vi "Cache.Result.Write.vi"(6 "Time (now)":timestamp, 7 "Idx":i32, 8 "error in (no error)":errorcluster, 9 "ProdComp":T1, 10 "Result in":T2) -> (0 "error out":errorcluster, 3 "File":string)   [LabVIEW 2016]
uses:
  Cache.TestSteps.Fglb.ResultData.ctl
  Database/ProdaNG/Controls/ProdaNG.ProcessResult.ctl
  Database/ProdaNG/Controls/ProdaNG.ProcessStepResult.ctl
  Database/ProdaNG/Controls/ProdaNG.TestStepResult.ctl
  Database/ProdaNG/Controls/ProdaNG.TestValueResult.ctl
  Cache.ProductComponent.Data.ctl
  Global/ApplicationGlobal.vi
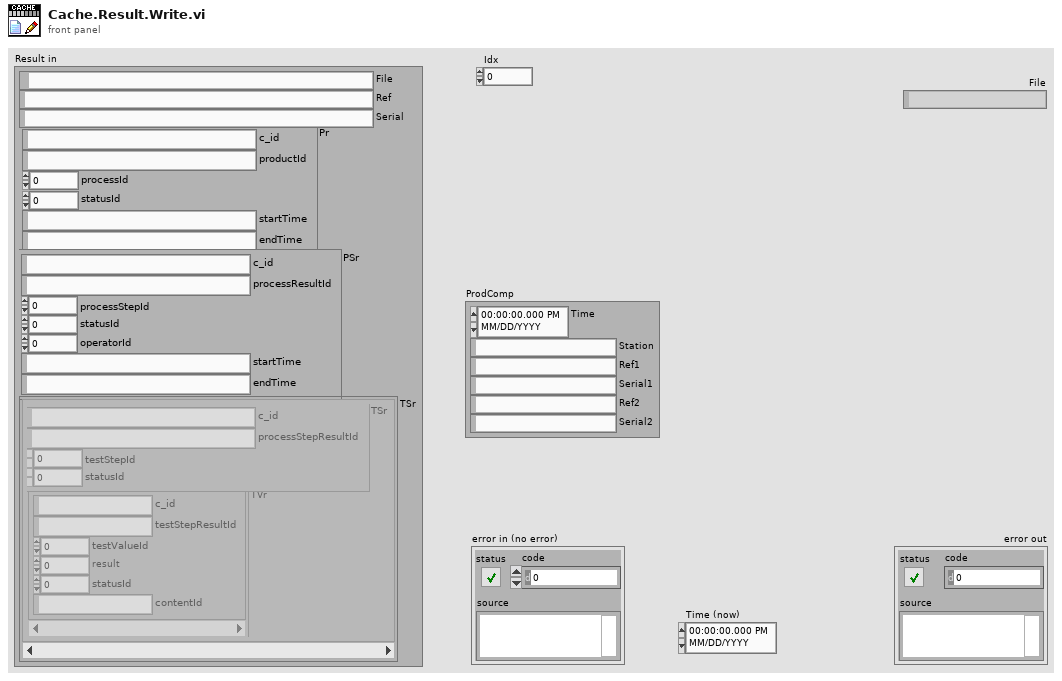
[diagram p1: front panel]
types:
  T1 = typedef "Cache.ProductComponent.Data.ctl" = cluster{"Time":timestamp, "Station":string, "Ref1":string, "Serial1":string, "Ref2":string, "Serial2":string}
  T2 = typedef "Cache.TestSteps.Fglb.ResultData.ctl" = cluster{"File":path, "Ref":string, "Serial":string, "Pr":T3, "PSr":T4, "TSr":cluster{"TSr":T5, "TVr":T6[]}[]}
  T3 = typedef "ProdaNG.ProcessResult.ctl" = cluster{"c_id":string, "productId":string, "processId":i32, "statusId":i32, "startTime":string, "endTime":string}
  T4 = typedef "ProdaNG.ProcessStepResult.ctl" = cluster{"c_id":string, "processResultId":string, "processStepId":i32, "statusId":i32, "operatorId":i32, "startTime":string, "endTime":string}
  T5 = typedef "ProdaNG.TestStepResult.ctl" = cluster{"c_id":string, "processStepResultId":string, "testStepId":i32, "statusId":i32}
  T6 = typedef "ProdaNG.TestValueResult.ctl" = cluster{"c_id":string, "testStepResultId":string, "testValueId":i32, "result":dbl, "statusId":i32, "contentId":string}
  T7 = enum16{"open", "open or create", "create or replace", "create", "open (read-only)"}
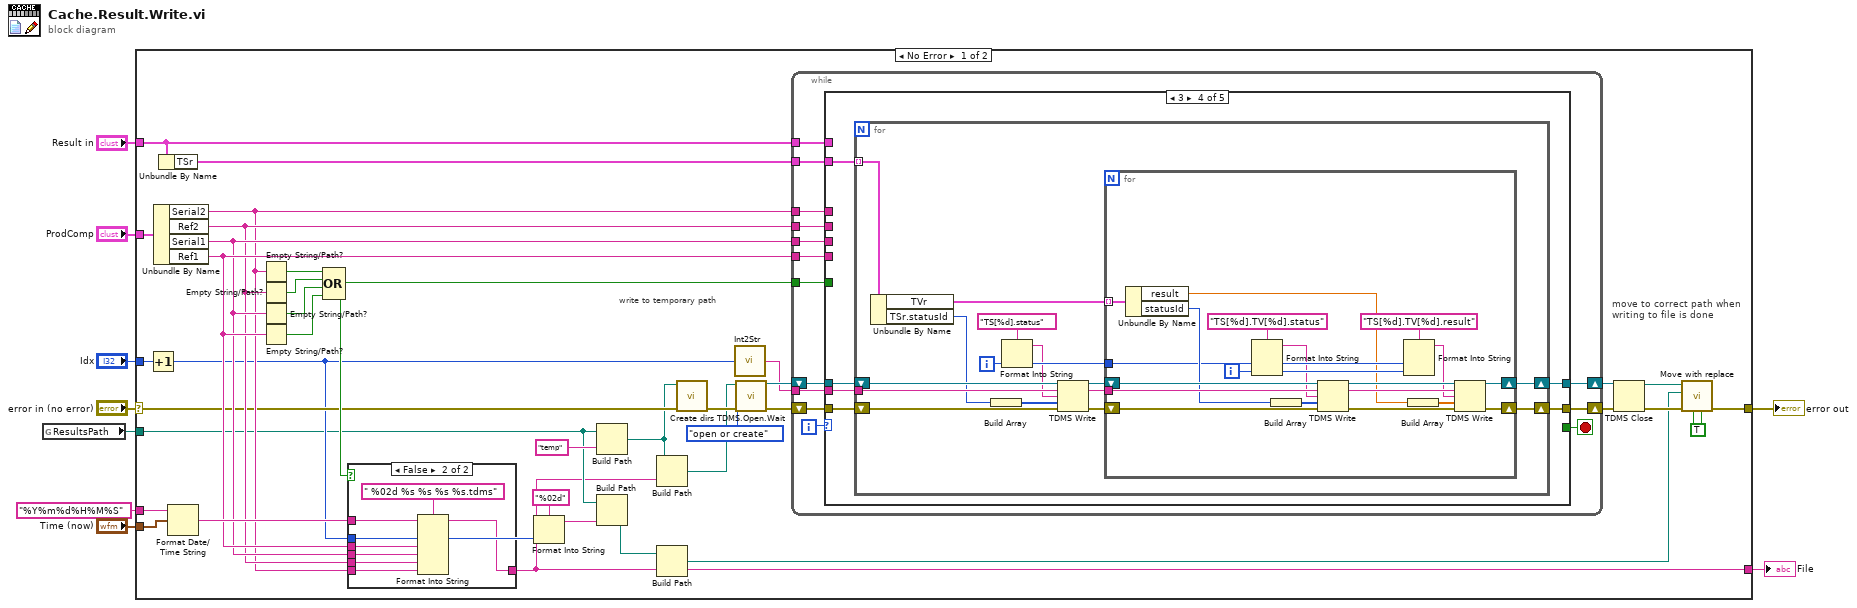
[diagram p0: block diagram]
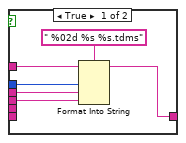
[diagram p2: hidden frame]
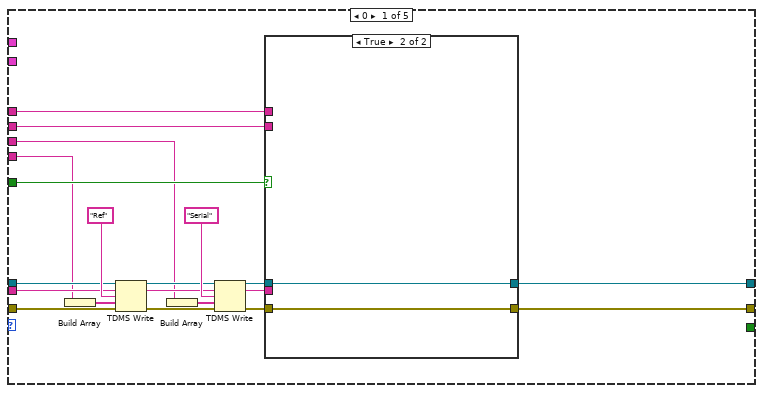
[diagram p3: hidden frame]
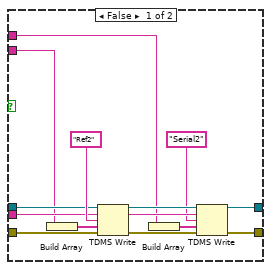
[diagram p4: hidden frame]
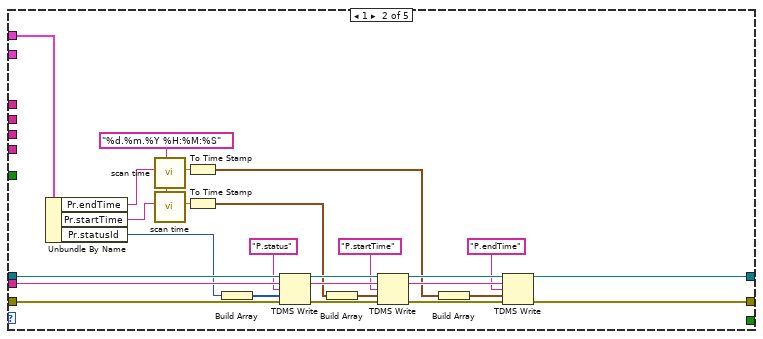
[diagram p5: hidden frame]
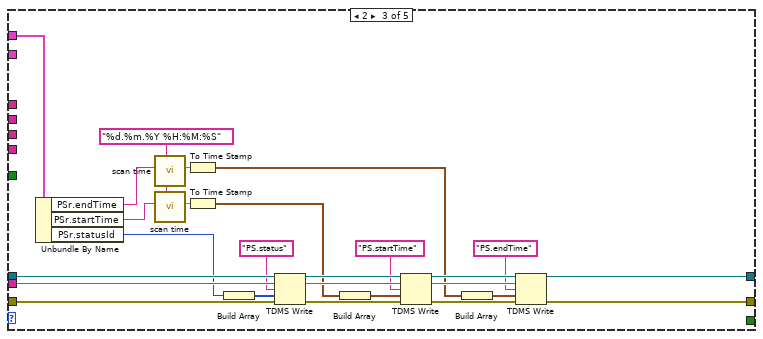
[diagram p6: hidden frame]
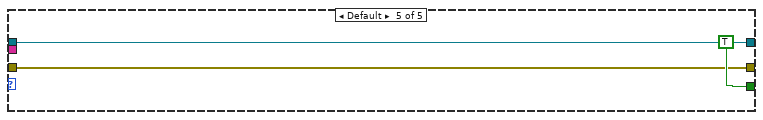
[diagram p7: hidden frame]
diagram:
  n1 = global read "ApplicationGlobal.vi" "ResultsPath"() -> (w4:path)
  n2 = case shown="No Error" "error in (no error)" {
    selector: "error in (no error)" -> [w25 w207]
    tunnel: "Result in" -> [w47 _]
    tunnel: [w20 w207] -> w9
    tunnel: "Idx" -> [w40 _]
    tunnel: "ProdComp" -> [w34 _]
    tunnel: w4 -> [w15 _]
    tunnel: "Time (now)" -> [w32 _]
    tunnel: "%Y%m%d%H%M%S" ("time format string (%c)") -> [w33 _]
    tunnel: [w12 _] -> w1
    frame No Error {
      w11 = TRUE ("create parent dirs (F)")
      # "move to correct path when \nwriting to file is done"
      # "write to temporary path"
      n3 = Increment(x=w40) -> (x+1=w23:i32)
      n4 = Unbundle By Name(w34) -> ("Serial2"=w26:string, "Ref2"=w27:string, "Serial1"=w28:string, "Ref1"=w29:string)
      n5 = Unbundle By Name(w47) -> ("TSr"=w43:cluster{"TSr":T5, "TVr":T6[]}[])
      n6 = Format Date/Time String(time format string (%c)=w33, seconds (now)=w32) -> (date/time string=w31:string)  [unwired: 1 in]
      n7 = Empty String/Path?(string/path=w26) -> (empty?=w38:bool)
      n8 = Empty String/Path?(string/path=w27) -> (empty?=w37:bool)
      n9 = Empty String/Path?(string/path=w28) -> (empty?=w36:bool)
      n10 = Empty String/Path?(string/path=w29) -> (empty?=w35:bool)
      n11 = Compound Arithmetic op=OR(w38, w37, w36, w35) -> (w30:bool)
      n12 = case shown="False" w30 {
        tunnel: [w48 w57] -> w12
        tunnel: w23 -> [w52 w54]
        tunnel: w31 -> [w49 w58]
        tunnel: w29 -> [w51 w60]
        tunnel: w28 -> [w50 w59]
        tunnel: w27 -> [_ w56]
        tunnel: w26 -> [_ w55]
        frame True {
          n13 = Format Into String(format string=" %02d %s %s.tdms" ("pattern"), initial string=w49, w52, w51, w50) -> (resulting string=w48:string)  [unwired: 1 in, 1 out]
        }
        frame False {
          n14 = Format Into String(format string=" %02d %s %s %s %s.tdms" ("pattern"), initial string=w58, w54, w60, w59, w56, w55) -> (resulting string=w57:string)  [unwired: 1 in, 1 out]
        }
      }
      n15 = Format Into String(format string="%02d" ("pattern"), w23) -> (resulting string=w22:string)  [unwired: 2 in, 1 out]
      n16 = Build Path(base path=w15, name or relative path="temp") -> (appended path=w13:path)
      n17 = Build Path(base path=w15, name or relative path=w22) -> (appended path=w16:path)
      n18 = Build Path(base path=w13, name or relative path=w12) -> (appended path=w14:path)
      n19 = Build Path(base path=w16, name or relative path=w12) -> (appended path=w10:path)
      n20 = call "Create dirs.vi"("error in (no error)"=w25, "deepest dir"=w13) -> ("error"=w24:errorcluster)  [unwired: 9 in]
      n21 = call "Int2Str.vi"("Numeric"=w23) -> ("string"=w39:string)
      n22 = call "TDMS.Open.Wait.vi"("error in (no error)"=w24, "operation (open read-only)"=T7."open or create" ("operation (0:open)"), "file path"=w14) -> ("error out"=w46:errorcluster, "tdms file out"=w41:refnum<k34>)  [unwired: 7 in]
      n23 = while {
        tunnel: w47 -> [w71]
        shift-right: [w72] -> w45
        shift-left: w41 -> [w75]
        shift-right: [w73] -> w44
        shift-left: w46 -> [w74]
        tunnel: w39 -> [w69]
        tunnel: w43 -> [w67]
        tunnel: w30 -> [w66]
        tunnel: w29 -> [w65]
        tunnel: w28 -> [w64]
        tunnel: w27 -> [w63]
        tunnel: w26 -> [w62]
        i -> [w70]
        stop <- w68 stop-if-true
        n24 = case shown="3" w70 {
          tunnel: w75 -> [w86 w137 w163 w166 w204]
          tunnel: w74 -> [w88 w136 w162 w168 w205]
          tunnel: [w82 w115 w140 w167 w205] -> w73
          tunnel: [w83 w116 w141 w165 w204] -> w72
          tunnel: w71 -> [_ w135 w161 _ _]
          tunnel: w69 -> [w87 w134 w160 w164 _]
          tunnel: [_ _ _ _ TRUE] -> w68
          tunnel: w67 -> [_ _ _ w169 _]
          tunnel: w66 -> [w80 _ _ _ _]
          tunnel: w65 -> [w79 _ _ _ _]
          tunnel: w64 -> [w78 _ _ _ _]
          tunnel: w63 -> [w77 _ _ _ _]
          tunnel: w62 -> [w76 _ _ _ _]
          frame 0 {
            n25 = Build Array(w79) -> (w89:string[])
            n26 = TDMS Write(0:w86, 5:w87, 7:"Ref", 9:w89, 11:w88) -> (4:w91:refnum<k34>, 6:w92:string, 15:w90:errorcluster)  [unwired: 1 in, 1 out]
            n27 = Build Array(w78) -> (w93:string[])
            n28 = TDMS Write(0:w91, 5:w92, 7:"Serial", 9:w93, 11:w90) -> (4:w85:refnum<k34>, 6:w81:string, 15:w84:errorcluster)  [unwired: 1 in, 1 out]
            n29 = case shown="True" w80 {
              tunnel: w85 -> [w102 w111]
              tunnel: w84 -> [w101 w110]
              tunnel: [w100 w111] -> w83
              tunnel: [w99 w110] -> w82
              tunnel: w81 -> [w98 _]
              tunnel: w77 -> [w97 _]
              tunnel: w76 -> [w96 _]
              frame False {
                n30 = Build Array(w97) -> (w109:string[])
                n31 = TDMS Write(0:w102, 5:w98, 7:"Ref2", 9:w109, 11:w101) -> (4:w107:refnum<k34>, 6:w106:string, 15:w108:errorcluster)  [unwired: 1 in, 1 out]
                n32 = Build Array(w96) -> (w105:string[])
                n33 = TDMS Write(0:w107, 5:w106, 7:"Serial2", 9:w105, 11:w108) -> (4:w100:refnum<k34>, 15:w99:errorcluster)  [unwired: 1 in, 2 out]
              }
              frame True {
              }
            }
          }
          frame 1 {
            w129 = "%d.%m.%Y %H:%M:%S" ("time format string")
            n34 = Unbundle By Name(w135) -> ("Pr.endTime"=w128:string, "Pr.startTime"=w131:string, "Pr.statusId"=w123:i32)
            n35 = call "scan time.vi"("time format string"=w129, "formatted time string"=w128) -> ("lv time (UTC)"=w130:dbl)  [unwired: 5 in, 4 out]
            n36 = call "scan time.vi"("time format string"=w129, "formatted time string"=w131) -> ("lv time (UTC)"=w132:dbl)  [unwired: 5 in, 4 out]
            n37 = To Time Stamp(1:w130) -> (0:w117:timestamp)
            n38 = To Time Stamp(1:w132) -> (0:w122:timestamp)
            n39 = Build Array(w123) -> (w133:i32[])
            n40 = TDMS Write(0:w137, 5:w134, 7:"P.status", 9:w133, 11:w136) -> (4:w126:refnum<k34>, 6:w125:string, 15:w127:errorcluster)  [unwired: 1 in, 1 out]
            n41 = Build Array(w122) -> (w124:timestamp[])
            n42 = TDMS Write(0:w126, 5:w125, 7:"P.startTime", 9:w124, 11:w127) -> (4:w118:refnum<k34>, 6:w119:string, 15:w120:errorcluster)  [unwired: 1 in, 1 out]
            n43 = Build Array(w117) -> (w121:timestamp[])
            n44 = TDMS Write(0:w118, 5:w119, 7:"P.endTime", 9:w121, 11:w120) -> (4:w116:refnum<k34>, 15:w115:errorcluster)  [unwired: 1 in, 2 out]
          }
          frame 2 {
            w155 = "%d.%m.%Y %H:%M:%S" ("time format string")
            n45 = Unbundle By Name(w161) -> ("PSr.endTime"=w154:string, "PSr.startTime"=w157:string, "PSr.statusId"=w149:i32)
            n46 = call "scan time.vi"("time format string"=w155, "formatted time string"=w154) -> ("lv time (UTC)"=w156:dbl)  [unwired: 5 in, 4 out]
            n47 = call "scan time.vi"("time format string"=w155, "formatted time string"=w157) -> ("lv time (UTC)"=w158:dbl)  [unwired: 5 in, 4 out]
            n48 = To Time Stamp(1:w156) -> (0:w143:timestamp)
            n49 = To Time Stamp(1:w158) -> (0:w148:timestamp)
            n50 = Build Array(w149) -> (w159:i32[])
            n51 = TDMS Write(0:w163, 5:w160, 7:"PS.status", 9:w159, 11:w162) -> (4:w152:refnum<k34>, 6:w151:string, 15:w153:errorcluster)  [unwired: 1 in, 1 out]
            n52 = Build Array(w148) -> (w150:timestamp[])
            n53 = TDMS Write(0:w152, 5:w151, 7:"PS.startTime", 9:w150, 11:w153) -> (4:w144:refnum<k34>, 6:w145:string, 15:w146:errorcluster)  [unwired: 1 in, 1 out]
            n54 = Build Array(w143) -> (w147:timestamp[])
            n55 = TDMS Write(0:w144, 5:w145, 7:"PS.endTime", 9:w147, 11:w146) -> (4:w141:refnum<k34>, 15:w140:errorcluster)  [unwired: 1 in, 2 out]
          }
          frame 3 {
            n56 = for {
              tunnel: w169 -> [w184] mode=indexing
              shift-right: [w175] -> w167
              shift-left: w168 -> [w183]
              shift-right: [w172] -> w165
              shift-left: w166 -> [w182]
              tunnel: w164 -> [w181]
              i -> [w177]
              n57 = Unbundle By Name(w184) -> ("TVr"=w178:T6[], "TSr.statusId"=w171:i32)
              n58 = Build Array(w171) -> (w180:i32[])
              n59 = Format Into String(format string="TS[%d].status", w177) -> (resulting string=w170:string)  [unwired: 2 in, 1 out]
              n60 = TDMS Write(0:w182, 5:w181, 7:w170, 9:w180, 11:w183) -> (4:w173:refnum<k34>, 6:w174:string, 15:w176:errorcluster)  [unwired: 1 in, 1 out]
              n61 = for {
                tunnel: w178 -> [w203] mode=indexing
                tunnel: w177 -> [w189]
                shift-right: [w194] -> w175
                shift-left: w176 -> [w202]
                tunnel: w174 -> [w200]
                shift-right: [w193] -> w172
                shift-left: w173 -> [w199]
                i -> [w188]
                n62 = Unbundle By Name(w203) -> ("result"=w186:dbl, "statusId"=w197:i32)
                n63 = Format Into String(format string="TS[%d].TV[%d].status", w189, w188) -> (resulting string=w187:string)  [unwired: 2 in, 1 out]
                n64 = Build Array(w197) -> (w198:i32[])
                n65 = TDMS Write(0:w199, 5:w200, 7:w187, 9:w198, 11:w202) -> (4:w192:refnum<k34>, 6:w191:string, 15:w195:errorcluster)  [unwired: 1 in, 1 out]
                n66 = Format Into String(format string="TS[%d].TV[%d].result", w189, w188) -> (resulting string=w185:string)  [unwired: 2 in, 1 out]
                n67 = Build Array(w186) -> (w196:dbl[])
                n68 = TDMS Write(0:w192, 5:w191, 7:w185, 9:w196, 11:w195) -> (4:w193:refnum<k34>, 15:w194:errorcluster)  [unwired: 1 in, 2 out]
              }
            }
          }
          frame Default {
          }
        }
      }
      n69 = TDMS Close(8:w44, 11:w45) -> (0:w21:errorcluster, 3:w19:path)
      n70 = call "Move with replace.vi"("create parent dirs (F)"=w11, "replace allowed (T)"=w11, "error in (no error)"=w21, "destination path"=w10, "source path"=w19) -> ("error"=w20:errorcluster)  [unwired: 6 in]
    }
    frame Error {
    }
  }
  "error out" <- w9
  "File" <- w1
